vi "main.vi"() -> ()   [LabVIEW 2018]
uses:
  Ctls/LoggingRate.ctl
  Ctls/MotorConfig.ctl
  Ctls/MotroConfigData.ctl
  Ctls/MagType.ctl
  Ctls/QueueData.ctl
  Ctls/State.ctl
  Ctls/CmdData.ctl
  Ctls/ConsumerLoopData.ctl
  Ctls/DisplayIndicator.ctl
  Ctls/DatabaseCmd.ctl
  Siemens S7 TCP v3_3 LV 8_5/Siemens S7 TCP v3_3 LV 8_5/S7 TCP API Library/S7 TCP.lvlib
panel:
  out "Motor#2_Speed":sgl(knob) caption="电机转速RPM" scale=0.0..50.0
  out "Motor#1_Speed":sgl(knob) caption="电机转速RPM" scale=0.05..50.0
  in  "Motor#2_Config":T1 caption="电机2配置"
  in  "Motor#2_Start?":bool caption="电机启动   1"
  in  "Motor#2_Direction":bool caption="电机方向\n正转          反转    1"
  in  "Motor#2_SpeedSet?":bool
  out "Motor#2_Current":dbl caption="电机电流   1" format="%1.1f"
  in  "Motor#2_SpeedSetting":dbl caption="电机速度设定 1" min=0.0 max=0.0 format="%.3f"
  out "Motor#2_Fault?":bool caption="故障指示 1"
  out "Motor#2_Running?":bool caption="电机运行指示"
  out "Motor#2_ConfigData":T2 caption="2#电机配置数据"
  out "Motor#1_ConfigData":T2 caption="1#电机配置数据"
  in  "Motor#1_Config":T1 caption="电机1配置"
  in  "Motor#1_SpeedSet?":bool
  in  "Log Length":i32=50
  in  "Logging Rate":T4=enum."5Hz"
  in  "Motor#3_Direction":bool caption="电机方向\n正转          反转"
  in  "sample interval (ms)":i32=100
  in  "Record":bool
  out "Speed Log to Display":string[][](table)
  out "Data Read":u8[][](array[numeric])
  out "Float Data Valid?":bool[](array[boolean])
  out "Bool Data Valid":bool
  in  "Stop Button":bool
  out "SpeedCurve":T5(graph) caption="实时显示"
  in  "ClearFault?":bool caption="故障复位"
  in  "Motor#3_SpeedSetting":dbl caption="电机速度设定 3" min=0.0 max=0.0 format="%.3g"
  in  "DualControl_Start?":bool caption="联动启动"
  out "Motor#2_Connected?":bool caption="通讯连接"
  out "Motor#1_Fault?":bool caption="故障指示 1"
  out "Motor#1_Running?":bool caption="电机运行指示"
  out "Motor#1_Connected？":bool caption="通讯连接    1"
  out "Motor#1_Current":dbl caption="电机电流   1" format="%1.1f"
  in  "Motor#1_SpeedSetting":dbl caption="电机速度设定 1" min=0.0 max=0.0 format="%.3f"
  in  "Motor#1_Start?":bool caption="电机启动   1"
  in  "Motor#1_Direction":bool caption="电机方向\n正转          反转    1"
  in  "SingleControl?":bool caption="单动            联动"
  # "1#大电机"
  # "2#大电机"
  # "A"
  # "A"
  # "RPS"
  # "RPS"
  # "RPS"
  # "注意：切换励磁请手动更改驱动器参数P50082,\n 当P50082=0时为永磁，P50082=1时为励磁！！"
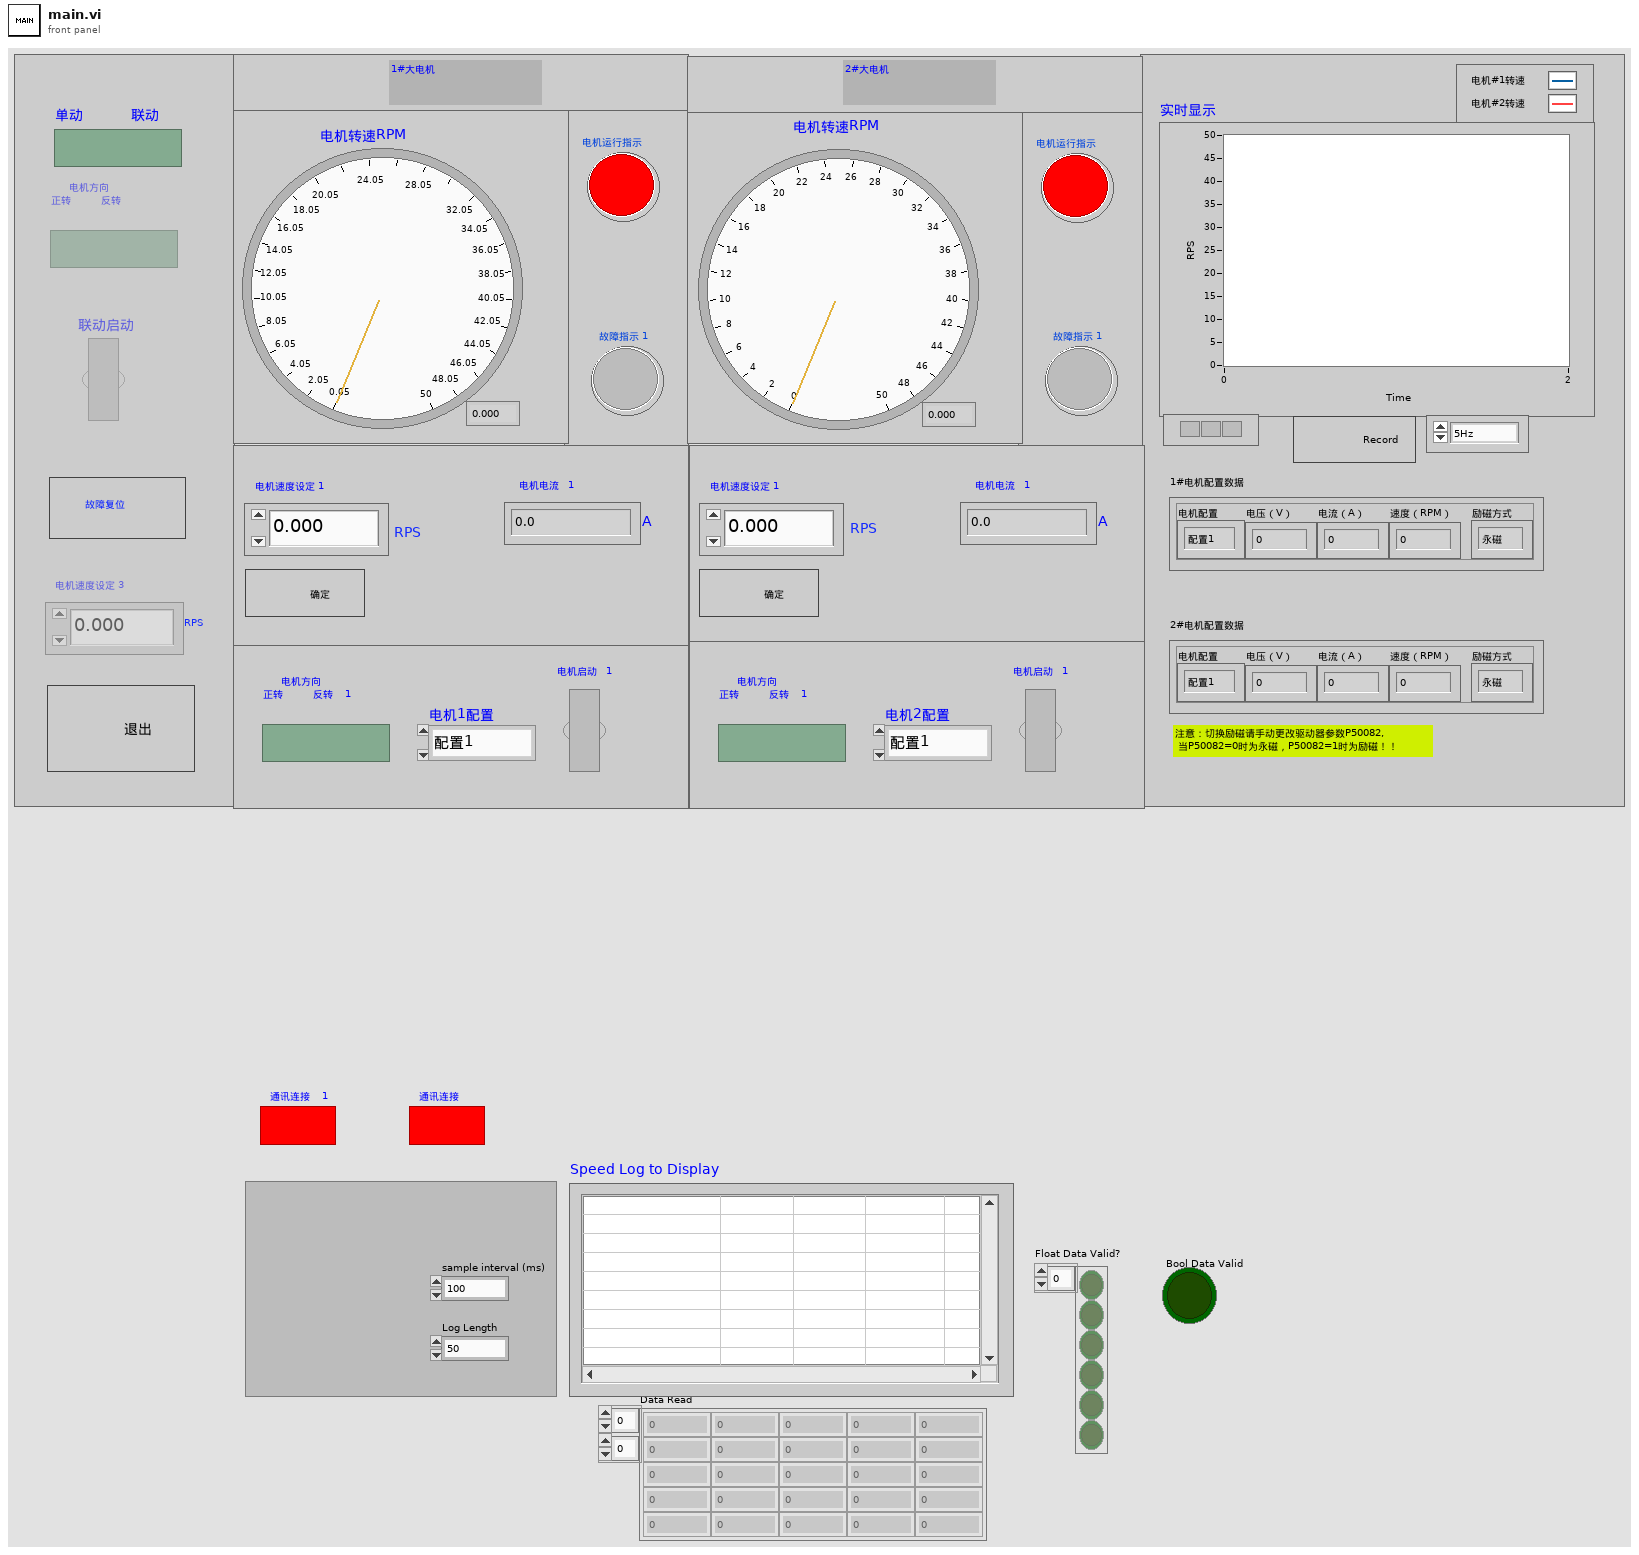
[diagram p1: front panel]
types:
  T1 = typedef "MotorConfig.ctl" = enum16{"配置1", "配置2", "配置3", "配置4"}
  T2 = typedef "MotroConfigData.ctl" = cluster{"电机配置":T1, "电压（V）":dbl, "电流（A）":dbl, "速度（RPM）":dbl, "励磁方式":T3}
  T3 = typedef "MagType.ctl" = enum16{"永磁", "励磁"}
  T4 = typedef "LoggingRate.ctl" = enum16{"1Hz", "2Hz", "5Hz", "10Hz", "20Hz"}
  T5 = cluster{"Motor Speed_1":sgl, "Motor Speed 2":sgl}
  T6 = typedef "ConsumerLoopData.ctl" = cluster{"CmdU16":u16, "Log File Path":path, "PLC Data":T7, "TCP Connection Ref":refnum<k5>, "Config File Path":path}
  T7 = typedef "DisplayIndicator.ctl" = cluster{"CommConnected_1":bool, "Run_1?":bool, "Fault_1?":bool, "CommConnected_2":bool, "Run_2?":bool, "Fault_2?":bool, "Motor Speed 2":sgl, "Motor Speed_1":sgl, "Motor Current_1":sgl, "Motor Current_2":sgl, "Motor1ConfigData":T2, "Motor2ConfigData":T2, "EmoStop_1?":bool}
  T8 = typedef "State.ctl" = enum16{"poll data command", "display update", "init", "send bool command", "send float command", "datalog", "error", "fix rating rpm 1", "fix rating rpm 2", "fix both rating rpm", "fix rating rpm all", "terminate", "log Motor Speed Setting"}
  T9 = typedef "QueueData.ctl" = cluster{"State":T8, "Command Data":T10}
  T10 = typedef "CmdData.ctl" = cluster{"Address Areas":u8, "Data Block #":u16, "Start Address (bytes)":u32, "Write Data Float":sgl, "Bit #":u16, "Write Data Boolean":bool}
  T11 = typedef "DatabaseCmd.ctl" = enum16{"Insert Table Title", "Add One Record", "Delete Record", "Get Table Records", "Clear"}
  T12 = enum8{"Enabled", "Disabled", "Disabled and Grayed Out"}
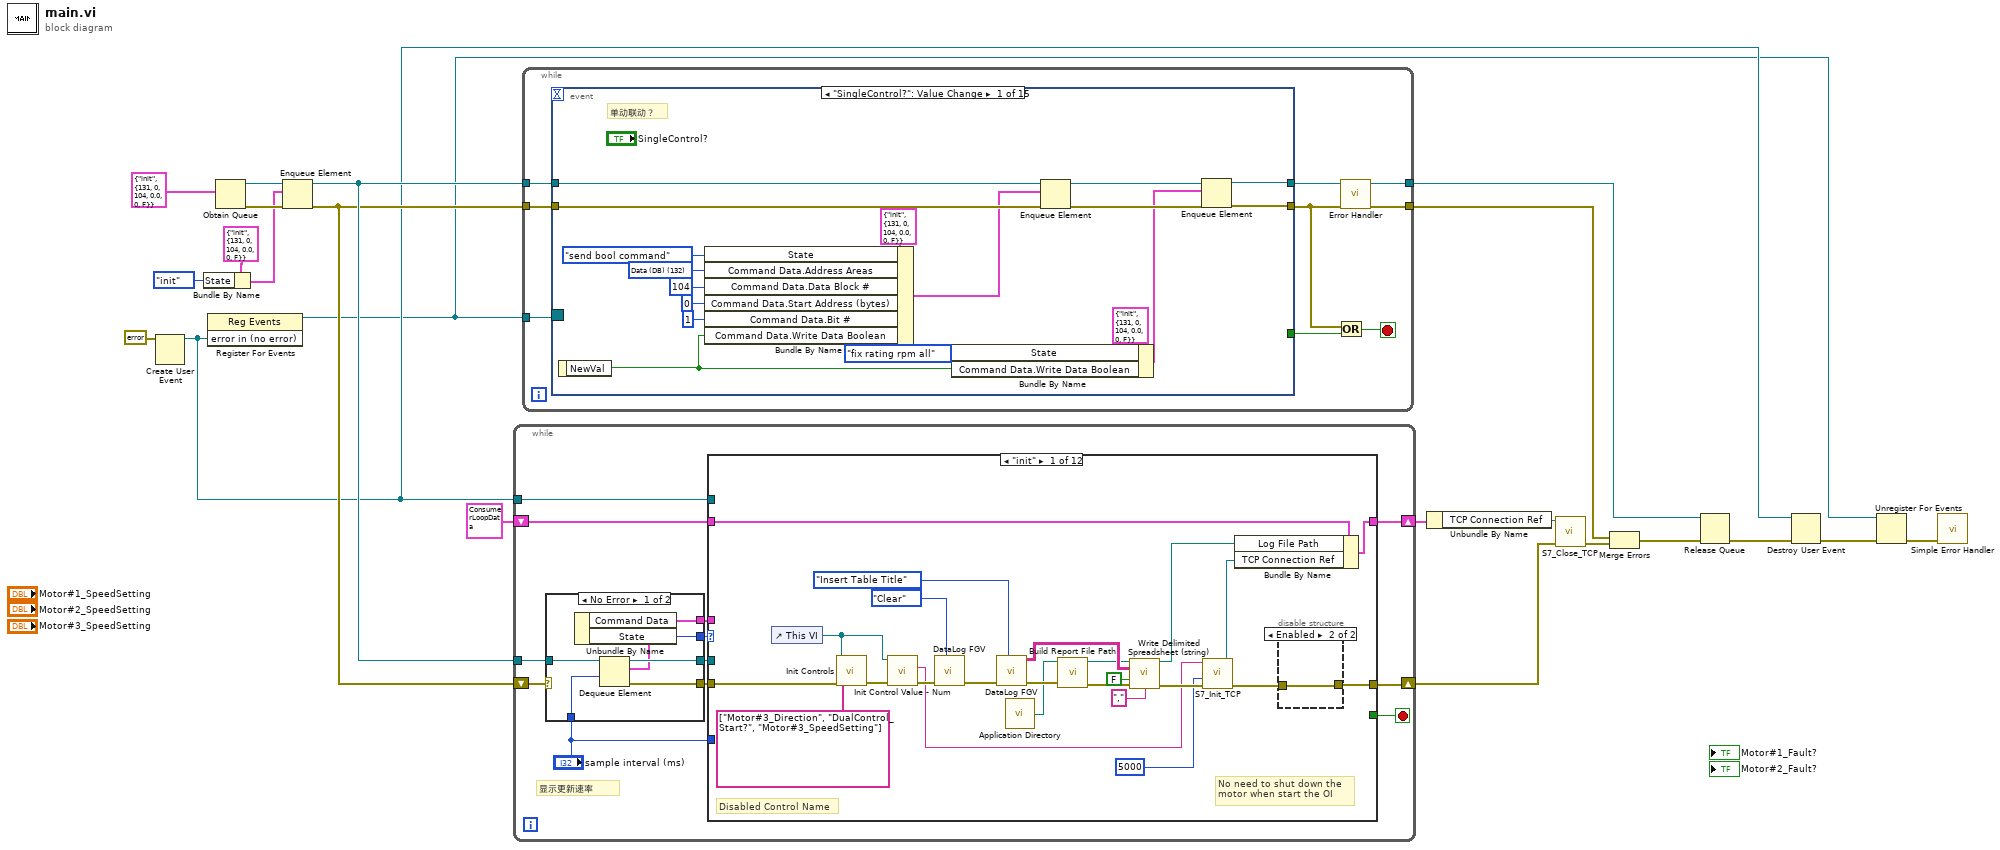
[diagram p0: block diagram]
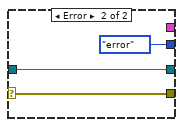
[diagram p2: hidden frame]
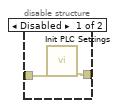
[diagram p3: hidden frame]
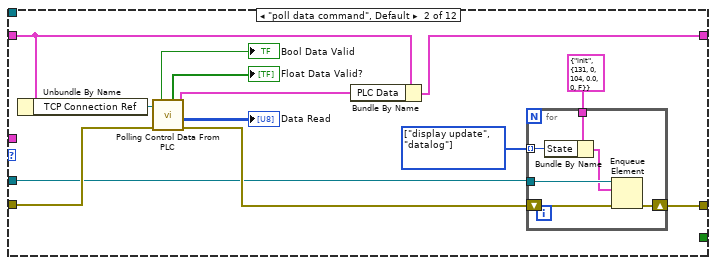
[diagram p4: hidden frame]
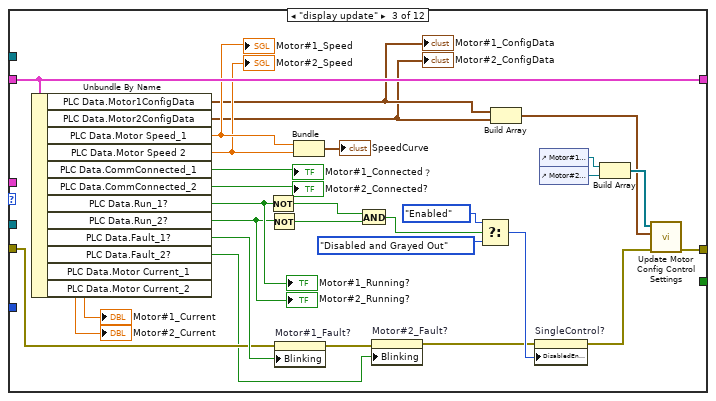
[diagram p5: hidden frame]
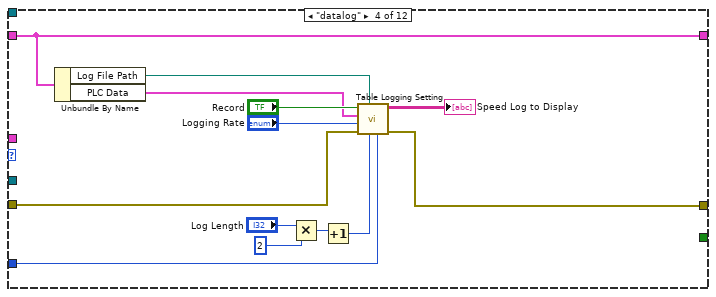
[diagram p6: hidden frame]
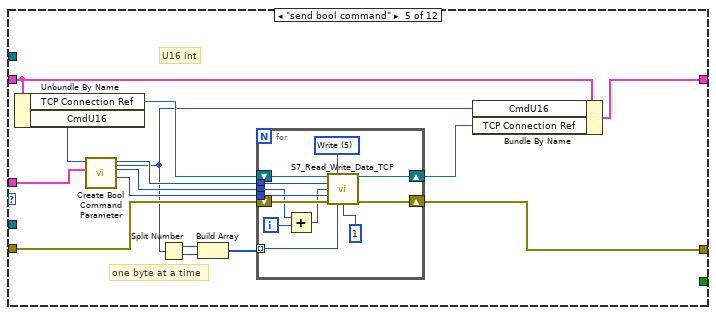
[diagram p7: hidden frame]
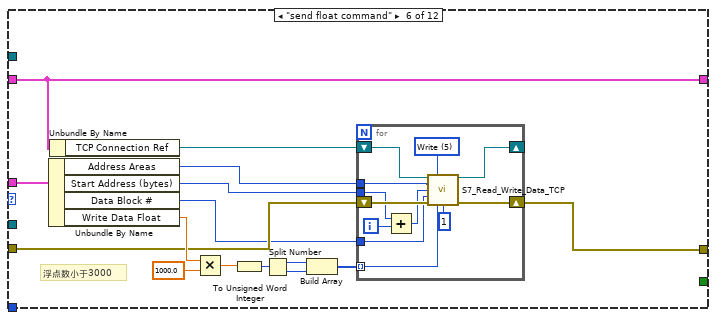
[diagram p8: hidden frame]
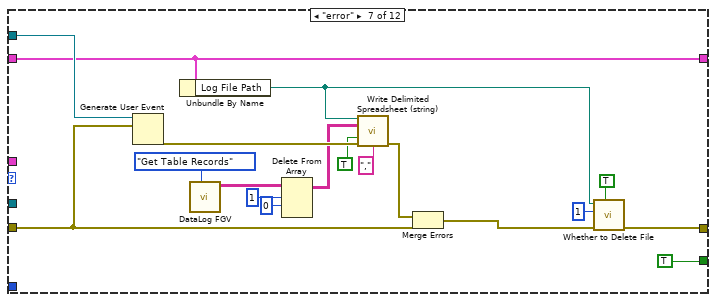
[diagram p9: hidden frame]
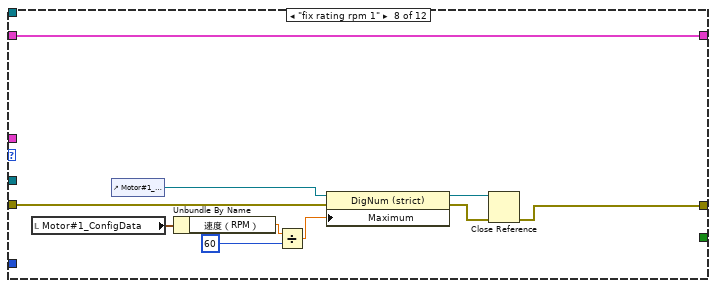
[diagram p10: hidden frame]
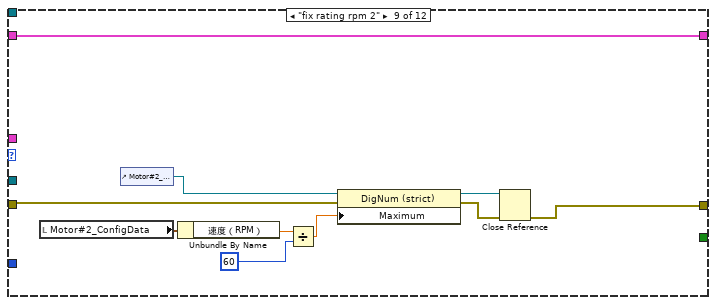
[diagram p11: hidden frame]
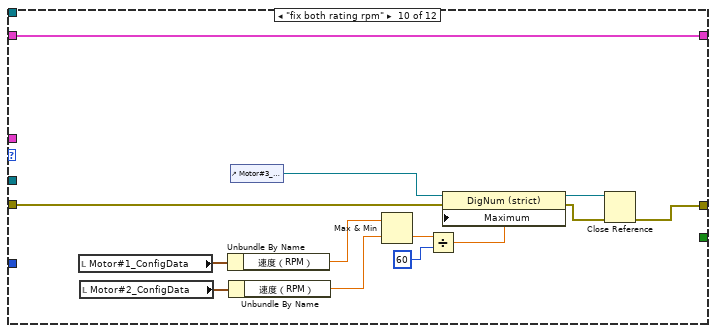
[diagram p12: hidden frame]
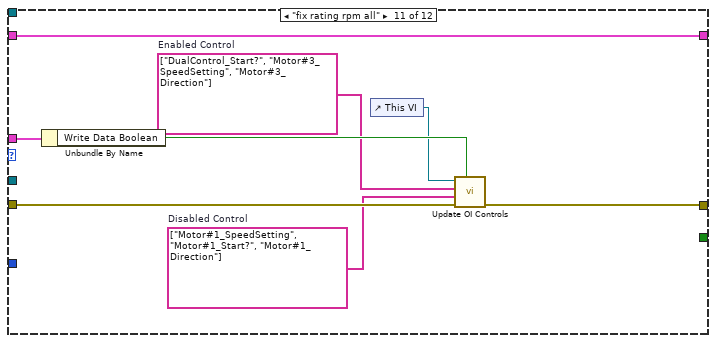
[diagram p13: hidden frame]
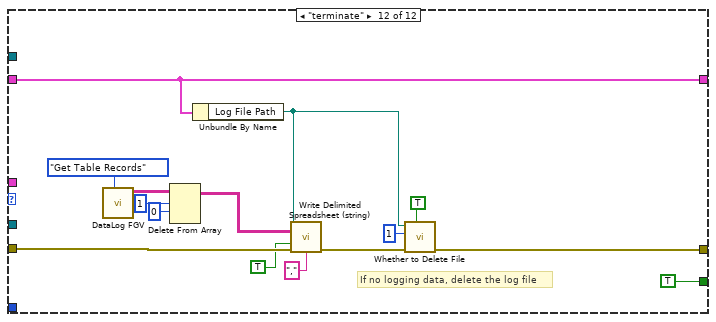
[diagram p14: hidden frame]
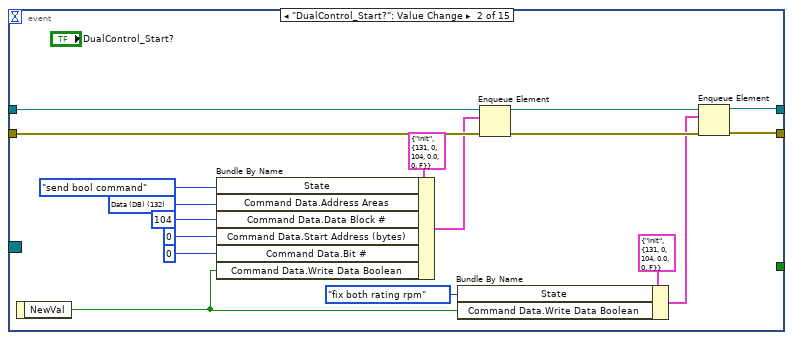
[diagram p15: hidden frame]
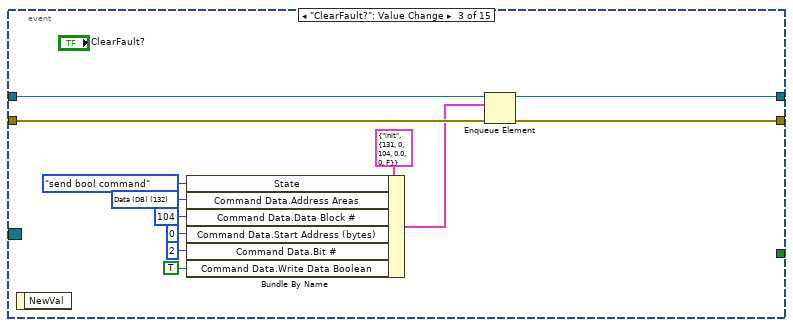
[diagram p16: hidden frame]
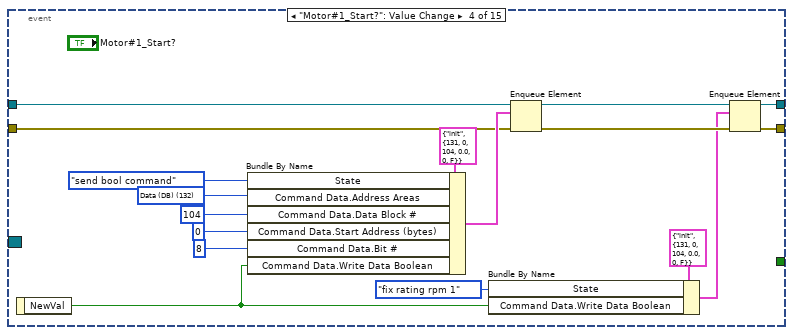
[diagram p17: hidden frame]
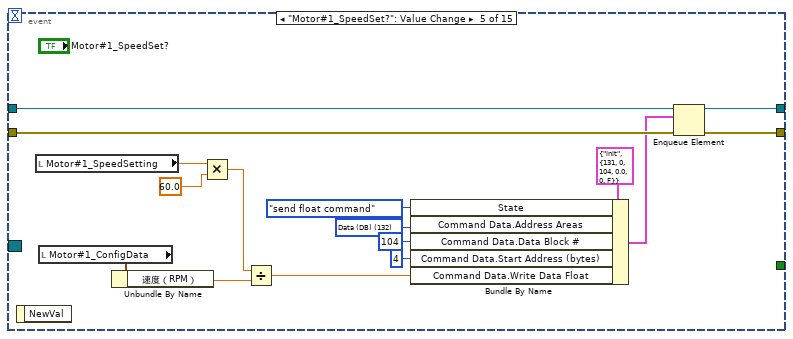
[diagram p18: hidden frame]
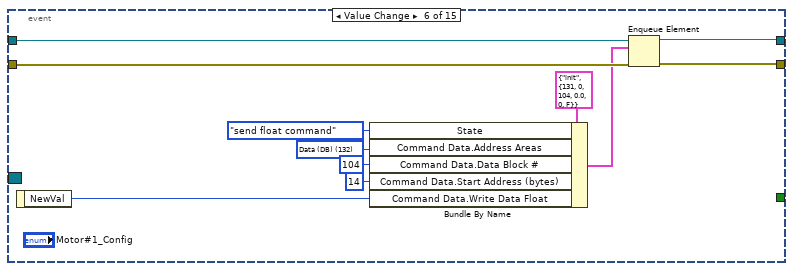
[diagram p19: hidden frame]
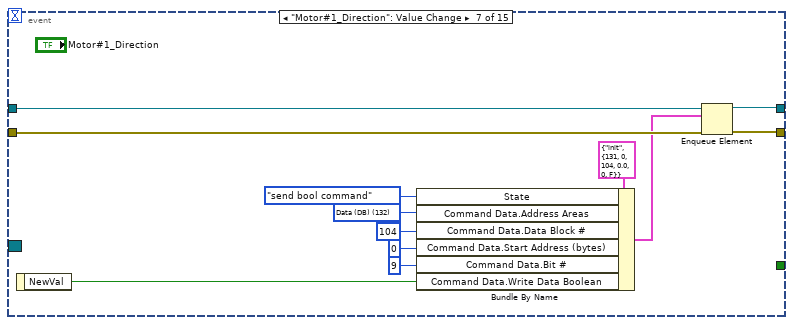
[diagram p20: hidden frame]
diagram:
  n1 = Create User Event(user event datatype=errorcluster {"status"=FALSE, "code"=0, "source"=""} ("error in (no error)")) -> (user event=w13:refnum<user-event>)  [unwired: 1 in, 1 out]
  n2 = Bundle By Name(cluster=T9 {"State"=enum."init", "Command Data"={"Address Areas"=131, "Data Block #"=0, "Start Address (bytes)"=104, "Write Data Float"=0.0, "Bit #"=0, "Write Data Boolean"=FALSE}} ("element"), "State"=State."init") -> (w15:T9)
  n3 = register-events(w13) -> (reference out=w11:refnum<event-registration>)  [unwired: 2 in, 1 out]
  n4 = Obtain Queue(element data type=T9 {"State"=enum."init", "Command Data"={"Address Areas"=131, "Data Block #"=0, "Start Address (bytes)"=104, "Write Data Float"=0.0, "Bit #"=0, "Write Data Boolean"=FALSE}} ("QData")) -> (queue out=w21:refnum<queue>, error out=w19:errorcluster)  [unwired: 4 in, 1 out]
  n5 = Enqueue Element(queue=w21, element=w15, error in (no error)=w19) -> (queue out=w20:refnum<queue>, error out=w18:errorcluster)  [unwired: 1 in, 1 out]
  n6 = while {
    tunnel: w20 -> [w26]
    tunnel: w13 -> [w29]
    shift-right: [w27] -> w10
    shift-left: w18 -> [w28]
    shift-right: [w24] -> w8
    shift-left: T6 {"CmdU16"=0, "Log File Path"=path "", "PLC Data"={"CommConnected_1"=FALSE, "Run_1?"=FALSE, "Fault_1?"=FALSE, "CommConnected_2"=FALSE, "Run_2?"=FALSE, "Fault_2?"=FALSE, "Motor Speed 2"=0.0, "Motor Speed_1"=0.0, "Motor Current_1"=0.0, "Motor Current_2"=0.0, "Motor1ConfigData"={"电机配置"=enum."配置1", "电压（V）"=0.0, "电流（A）"=0.0, "速度（RPM）"=0.0, "励磁方式"=enum."永磁"}, "Motor2ConfigData"={"电机配置"=enum."配置1", "电压（V）"=0.0, "电流（A）"=0.0, "速度（RPM）"=0.0, "励磁方式"=enum."永磁"}, "EmoStop_1?"=FALSE}, "TCP Connection Ref"=refnum, "Config File Path"=path ""} ("Consumer Loop Data") -> [w25]
    stop <- w30 stop-if-true
    # "显示更新速率"
    n7 = case shown="No Error" w28 {
      selector: w28 -> [_ w44]
      tunnel: [w41 w43] -> w34
      tunnel: [w40 w44] -> w33
      tunnel: [w38 State."error" ("State")] -> w32
      tunnel: [w37 _] -> w31
      tunnel: w26 -> [w36 w43]
      tunnel: "sample interval (ms)" -> [w35 _]
      frame No Error {
        n8 = Dequeue Element(queue=w36, timeout in ms (-1)=w35) -> (queue out=w41:refnum<queue>, element=w39:T9, error out=w40:errorcluster)  [unwired: 1 in, 1 out]
        n9 = Unbundle By Name(w39) -> ("Command Data"=w37:T10, "State"=w38:T8)
      }
      frame Error {
      }
    }
    n10 = case shown="\"init\"" w32 {
      tunnel: w34 -> [_ w78 _ _ _ _ _ _ _ _ _ _]
      tunnel: w33 -> [w53 w84 w108 w130 w147 w168 w202 w212 w222 w237 w243 w255]
      tunnel: [w55 w79 w112 w129 w139 w162 w188 w206 w215 w226 w244 w249] -> w27
      tunnel: w31 -> [_ _ _ _ w146 w174 _ _ _ _ w245 _]
      tunnel: [_ _ _ _ _ _ TRUE ("Data Valid") _ _ _ _ TRUE ("Data Valid")] -> w30
      tunnel: w29 -> [_ _ _ _ _ _ w203 _ _ _ _ _]
      tunnel: w25 -> [w52 w75 w111 w121 w136 w160 w192 w205 w216 w225 w242 w251]
      tunnel: [w49 w73 w111 w121 w133 w160 w192 w205 w216 w225 w242 w251] -> w24
      tunnel: "sample interval (ms)" -> [_ _ _ w120 _ _ _ _ _ _ _ _]
      frame "init" {
        # "Disabled Control Name"
        # "No need to shut down the \nmotor when start the OI"
        n11 = control-ref of="This VI"() -> (w46:refnum<vi>)
        n12 = call "Init Controls.vi"("error in"=w53, "Disabled Controls"=string[] ["Motor#3_Direction", "DualControl_Start?", "Motor#3_SpeedSetting"], "VI ref"=w46) -> ("error out"=w48:errorcluster)  [unwired: 8 in]
        n13 = call "Init Control Value - Num.vi"("error in (no error)"=w48, "This VI"=w46) -> ("error out"=w47:errorcluster, "PLC IP"=w45:string)  [unwired: 7 in, 1 out]
        n14 = call "DataLog FGV.vi"("Method"=DatabaseCmd."Clear", "error in (no error)"=w47) -> ("error out"=w68:errorcluster)  [unwired: 7 in, 2 out]
        n15 = call "DataLog FGV.vi"("Method"=DatabaseCmd."Insert Table Title", "error in (no error)"=w68) -> ("error out"=w67:errorcluster, "Speed Log"=w66:string[][])  [unwired: 7 in, 1 out]
        n16 = call <vilib>:"Application Directory.vi"() -> ("Application Directory"=w60:path)
        n17 = call "Build Report File Path.vi"("error in (no error)"=w67, "File Path in"=w60) -> ("error out"=w64:errorcluster, "Report Path out"=w65:path)  [unwired: 8 in]
        n18 = call "Write Delimited Spreadsheet (string).vi"("Path"=w65, "2D data"=w66, "append to file?"=FALSE ("append to file? (new file:F)"), "error in"=w64, "delimiter (\\t)"="," ("delimiter (\\t)")) -> ("path"=w51:path, "error out"=w58:errorcluster)  [unwired: 9 in]
        n19 = call "S7_Init_TCP.vi"("error in"=w58, "Connection Timeout"=u32 5000, "IP Address"=w45) -> ("error out"=w56:errorcluster, "TCP Connection Ref"=w50:refnum<k5>)  [unwired: 2 in, 5 out]
        n20 = Bundle By Name(cluster=w52, "Log File Path"=w51, "TCP Connection Ref"=w50) -> (w49:T6)
        n21 = disable-structure shown="Enabled" {
          disable-tunnel: w56 -> [w70 w71]
          disable-tunnel: [w69 w71] -> w55
          frame Disabled {
            n22 = call "Init PLC Settings.vi"("error in"=w70) -> ("error out"=w69:errorcluster)  [unwired: 9 in, 1 out]
          }
          frame Enabled {
          }
        }
      }
      frame "poll data command", Default {
        w76 = T8[] [enum."display update", enum."datalog"] items=["poll data command", "display update", "init", "send bool command", "send float command", "datalog", "error", "fix rating rpm 1", "fix rating rpm 2", "fix both rating rpm", "fix rating rpm all", "terminate", "log Motor Speed Setting"]
        n23 = Unbundle By Name(w75) -> ("TCP Connection Ref"=w72:refnum<k5>)
        n24 = call "Polling Control Data From PLC.vi"("error in (no error)"=w84, "TCP Network Connection in"=w72) -> ("error out"=w80:errorcluster, "Data Read"=→"Data Read":u8[][], "PLC Data out"=w74:T7, "Bool Data Valid"=→"Bool Data Valid":bool, "Float Data Valid?"=→"Float Data Valid?":bool[])  [unwired: 2 in, 3 out]
        n25 = Bundle By Name(cluster=w75, "PLC Data"=w74) -> (w73:T6)
        n26 = for {
          tunnel: w78 -> [w88]
          shift-right: [w89] -> w79
          shift-left: w80 -> [w90]
          tunnel: T9 {"State"=enum."init", "Command Data"={"Address Areas"=131, "Data Block #"=0, "Start Address (bytes)"=104, "Write Data Float"=0.0, "Bit #"=0, "Write Data Boolean"=FALSE}} ("QData") -> [w86]
          tunnel: w76 -> [w85] mode=indexing
          n27 = Bundle By Name(cluster=w86, "State"=w85) -> (w87:T9)
          n28 = Enqueue Element(queue=w88, element=w87, error in (no error)=w90) -> (error out=w89:errorcluster)  [unwired: 1 in, 2 out]
        }
      }
      frame "display update" {
        n29 = Unbundle By Name(w111) -> ("PLC Data.Motor1ConfigData"=w96:T2, "PLC Data.Motor2ConfigData"=w95:T2, "PLC Data.Motor Speed_1"=w98:sgl, "PLC Data.Motor Speed 2"=w97:sgl, "PLC Data.CommConnected_1"=→"Motor#1_Connected？":bool, "PLC Data.CommConnected_2"=→"Motor#2_Connected?":bool, "PLC Data.Run_1?"=w100:bool, "PLC Data.Run_2?"=w99:bool, "PLC Data.Fault_1?"=w109:bool, "PLC Data.Fault_2?"=w107:bool, "PLC Data.Motor Current_1"=→"Motor#1_Current":sgl, "PLC Data.Motor Current_2"=→"Motor#2_Current":sgl)
        "Motor#1_Running?" <- w100
        "Motor#2_Running?" <- w99
        "Motor#1_ConfigData" <- w96
        "Motor#2_ConfigData" <- w95
        "Motor#1_Speed" <- w98
        "Motor#2_Speed" <- w97
        n30 = Not(x=w100) -> (.not. x?=w118:bool)
        n31 = Not(x=w99) -> (.not. x?=w119:bool)
        n32 = property on="Motor#1_Fault?" class="Bool (strict)"(error in=w108, "Blinking"=w109) -> (error out=w106:errorcluster)  [unwired: 1 in, 1 out]
        n33 = Bundle("Motor Speed_1"=w98, "Motor Speed 2"=w97) -> (→"SpeedCurve":T5)  [unwired: 1 in]
        n34 = And(x=w118, y=w119) -> (x .and. y?=w117:bool)
        n35 = property on="Motor#2_Fault?" class="Bool (strict)"(error in=w106, "Blinking"=w107) -> (error out=w105:errorcluster)  [unwired: 1 in, 1 out]
        n36 = Select(t=T12."Enabled" ("Disabled"), s=w117, f=T12."Disabled and Grayed Out" ("Disabled")) -> (s? t:f=w114:T12)
        n37 = Build Array(w96, w95) -> (w91:T2[])
        n38 = property on="SingleControl?" class="Bool (strict)"(error in=w105, "DisabledEnum"=w114) -> (error out=w113:errorcluster)  [unwired: 1 in, 1 out]
        n39 = control-ref of="Motor#1_Config"() -> (w94:refnum<vi>)
        n40 = control-ref of="Motor#2_Config"() -> (w93:refnum<vi>)
        n41 = Build Array(w94, w93) -> (w92:refnum<vi>[])
        n42 = call "Update Motor Config Control Settings.vi"("error in (no error)"=w113, "Motor Config Data"=w91, "Motor Config Refs"=w92) -> ("error out"=w112:errorcluster)  [unwired: 8 in]
      }
      frame "datalog" {
        n43 = Unbundle By Name(w121) -> ("Log File Path"=w123:path, "PLC Data"=w122:T7)
        n44 = Multiply(x="Log Length", y=2) -> (x*y=w125:i32)
        n45 = Increment(x=w125) -> (x+1=w124:i32)
        n46 = call "Table Logging Setting.vi"("sample interval (ms)"=w120, "Log Length"=w124, "Log File path"=w123, "error in (no error)"=w130, "Logging Rate"="Logging Rate", "Data In"=w122, "Record"="Record") -> ("error out"=w129:errorcluster, "Speed Log to Display"=→"Speed Log to Display":string[][])  [unwired: 3 in]
      }
      frame "send bool command" {
        # "one byte at a time"
        # "U16 int"
        n47 = Unbundle By Name(w136) -> ("TCP Connection Ref"=w137:refnum<k5>, "CmdU16"=w138:u16)
        n48 = call "Create Bool Command Parameter.vi"("Command Data"=w146, "Cmd U16"=w138) -> ("Data Block #"=w143:u16, "Start Address (bytes)"=w144:u32, "Address Areas"=w145:u8, "Cmd U16 out"=w135:u16)  [unwired: 6 in]
        n49 = Split Number(x=w135) -> (hi(x)=w141:u8, lo(x)=w140:u8)
        n50 = Build Array(w141, w140) -> (w142:u8[])
        n51 = for {
          tunnel: w145 -> [w155]
          tunnel: w144 -> [w149]
          tunnel: w143 -> [w154]
          shift-right: [w156] -> w134
          shift-left: w137 -> [w159]
          shift-right: [w152] -> w139
          shift-left: w147 -> [w158]
          tunnel: w142 -> [w151] mode=indexing
          i -> [w150]
          w157 = u8 5 items=["Read"=4, "Write"=5] ("Read / Write")
          n52 = Add(x=w149, y=w150) -> (x+y=w148:u32)
          n53 = call "S7_Read_Write_Data_TCP.vi"("TCP Connection Ref"=w159, "Read / Write"=w157, "Address Areas"=w155, "Start Address (bytes)"=w148, "Data Block #"=w154, "error in"=w158, "Write Data"=w151, "Length (bytes)"=u16 1) -> ("TCP Connection Ref Out"=w156:refnum<k5>, "error out"=w152:errorcluster)  [unwired: 2 in, 4 out]
        }
        n54 = Bundle By Name(cluster=w136, "CmdU16"=w135, "TCP Connection Ref"=w134) -> (w133:T6)
      }
      frame "send float command" {
        # "浮点数小于3000"
        n55 = Unbundle By Name(w174) -> ("Address Areas"=w167:u8, "Start Address (bytes)"=w166:u32, "Data Block #"=w165:u16, "Write Data Float"=w173:sgl)
        n56 = Unbundle By Name(w160) -> ("TCP Connection Ref"=w161:refnum<k5>)
        n57 = Multiply(x=w173, y=sgl 1000.0) -> (x*y=w171:sgl)
        n58 = To Unsigned Word Integer(number=w171) -> (unsigned 16bit integer=w170:u16)
        n59 = Split Number(x=w170) -> (hi(x)=w164:u8, lo(x)=w163:u8)
        n60 = Build Array(w164, w163) -> (w169:u8[])
        n61 = for {
          shift-right: [w183] -> _
          shift-left: w161 -> [w186]
          shift-right: [w181] -> w162
          shift-left: w168 -> [w185]
          tunnel: w169 -> [w178] mode=indexing
          tunnel: w167 -> [w177]
          tunnel: w166 -> [w176]
          tunnel: w165 -> [w175]
          i -> [w180]
          w184 = u8 5 items=["Read"=4, "Write"=5] ("Read / Write")
          n62 = Add(x=w176, y=w180) -> (x+y=w179:u32)
          n63 = call "S7_Read_Write_Data_TCP.vi"("TCP Connection Ref"=w186, "Read / Write"=w184, "Address Areas"=w177, "Start Address (bytes)"=w179, "Data Block #"=w175, "error in"=w185, "Write Data"=w178, "Length (bytes)"=u16 1) -> ("TCP Connection Ref Out"=w183:refnum<k5>, "error out"=w181:errorcluster)  [unwired: 2 in, 4 out]
        }
      }
      frame "error" {
        n64 = Generate User Event(user event=w203, event data cluster=w202) -> (error out=w201:errorcluster)  [unwired: 2 in, 1 out]
        n65 = Unbundle By Name(w192) -> ("Log File Path"=w187:path)
        n66 = call "DataLog FGV.vi"("Method"=DatabaseCmd."Get Table Records") -> ("Speed Log"=w197:string[][])  [unwired: 8 in, 2 out]
        n67 = Delete From Array(array=w197, length=1, index (row)=0) -> (array with subset deleted=w194:string[][])  [unwired: 1 in, 1 out]
        n68 = call "Write Delimited Spreadsheet (string).vi"("Path"=w187, "2D data"=w194, "append to file?"=TRUE ("append to file? (new file:F)"), "error in"=w201, "delimiter (\\t)"="," ("delimiter (\\t)")) -> ("error out"=w200:errorcluster)  [unwired: 9 in, 1 out]
        n69 = Merge Errors(w200, w202) -> (w189:errorcluster)
        n70 = call "Whether to Delete File.vi"("Del Log file?"=TRUE, "error in (no error)"=w189, "Number of lines"=1, "File path"=w187) -> ("error out"=w188:errorcluster)  [unwired: 7 in]
      }
      frame "fix rating rpm 1" {
        n71 = local read "Motor#1_ConfigData"() -> (w208:T2)
        n72 = control-ref of="Motor#1_SpeedSetting"() -> (w211:refnum<vi>)
        n73 = Unbundle By Name(w208) -> ("速度（RPM）"=w207:dbl)
        n74 = Divide(x=w207, y=u16 60) -> (x/y=w213:dbl)
        n75 = property class="DigNum (strict)"(reference=w211, error in=w212, "Maximum"=w213) -> (reference out=w209:refnum<vi>, error out=w210:errorcluster)
        n76 = Close Reference(reference=w209, error in (no error)=w210) -> (error out=w206:errorcluster)
      }
      frame "fix rating rpm 2" {
        n77 = local read "Motor#2_ConfigData"() -> (w219:T2)
        n78 = control-ref of="Motor#2_SpeedSetting"() -> (w217:refnum<vi>)
        n79 = Unbundle By Name(w219) -> ("速度（RPM）"=w218:dbl)
        n80 = Divide(x=w218, y=u16 60) -> (x/y=w223:dbl)
        n81 = property class="DigNum (strict)"(reference=w217, error in=w222, "Maximum"=w223) -> (reference out=w220:refnum<vi>, error out=w221:errorcluster)
        n82 = Close Reference(reference=w220, error in (no error)=w221) -> (error out=w215:errorcluster)
      }
      frame "fix both rating rpm" {
        n83 = local read "Motor#1_ConfigData"() -> (w228:T2)
        n84 = local read "Motor#2_ConfigData"() -> (w230:T2)
        n85 = Unbundle By Name(w228) -> ("速度（RPM）"=w227:dbl)
        n86 = Unbundle By Name(w230) -> ("速度（RPM）"=w229:dbl)
        n87 = control-ref of="Motor#3_SpeedSetting"() -> (w236:refnum<vi>)
        n88 = Max & Min(x=w227, y=w229) -> (min(x,y)=w233:dbl)  [unwired: 1 out]
        n89 = Divide(x=w233, y=u16 60) -> (x/y=w231:dbl)
        n90 = property class="DigNum (strict)"(reference=w236, error in=w237, "Maximum"=w231) -> (reference out=w234:refnum<vi>, error out=w235:errorcluster)
        n91 = Close Reference(reference=w234, error in (no error)=w235) -> (error out=w226:errorcluster)
      }
      frame "fix rating rpm all" {
        w239 = string[] ["DualControl_Start?", "Motor#3_SpeedSetting", "Motor#3_Direction"]  # Enabled Control
        w238 = string[] ["Motor#1_SpeedSetting", "Motor#1_Start?", "Motor#1_Direction"]  # Disabled Control
        n92 = Unbundle By Name(w245) -> ("Write Data Boolean"=w241:bool)
        n93 = control-ref of="This VI"() -> (w240:refnum<vi>)
        n94 = call "Update OI Controls.vi"("ControlBoth?"=w241, "error in (no error)"=w243, "Disabled Controls"=w238, "Enabled Controls"=w239, "VI Ref"=w240) -> ("error out"=w244:errorcluster)  [unwired: 6 in]
      }
      frame "terminate" {
        # "If no logging data, delete the log file"
        n95 = call "DataLog FGV.vi"("Method"=DatabaseCmd."Get Table Records") -> ("Speed Log"=w258:string[][])  [unwired: 8 in, 2 out]
        n96 = Delete From Array(array=w258, length=1, index (row)=0) -> (array with subset deleted=w254:string[][])  [unwired: 1 in, 1 out]
        n97 = Unbundle By Name(w251) -> ("Log File Path"=w248:path)
        n98 = call "Write Delimited Spreadsheet (string).vi"("Path"=w248, "2D data"=w254, "append to file?"=TRUE ("append to file? (new file:F)"), "error in"=w255, "delimiter (\\t)"="," ("delimiter (\\t)")) -> ("error out"=w250:errorcluster)  [unwired: 9 in, 1 out]
        n99 = call "Whether to Delete File.vi"("Del Log file?"=TRUE, "error in (no error)"=w250, "Number of lines"=1, "File path"=w248) -> ("error out"=w249:errorcluster)  [unwired: 7 in]
      }
    }
  }
  n100 = while {
    tunnel: w20 -> [w269]
    tunnel: w18 -> [w268]
    tunnel: w11 -> [w267]
    tunnel: [w262] -> w5
    tunnel: [w261] -> w4
    stop <- w265 stop-if-true
    n101 = event shown="[0] \"SingleControl?\": Value Change" {
      selector: w267 -> [_ _ _ _ _ _ _ _ _ _ _ _ _ _ _]
      dyn-events: _ -> [_ _ _ _ _ _ _ _ _ _ _ _ _ _ _]
      timeout: _ -> [_ _ _ _ _ _ _ _ _ _ _ _ _ _ _]
      tunnel: [_ _ _ _ _ _ _ _ _ _ _ _ _ TRUE ("Stop Button") TRUE ("Stop Button")] -> w266
      tunnel: w269 -> [w286 w302 w315 w324 w347 w358 w370 w397 w409 w421 w437 w449 w466 w470 w479]
      tunnel: w268 -> [w285 w301 w314 w323 w345 w356 w368 w396 w407 w419 w436 w447 w465 w468 w478]
      tunnel: [w278 w296 w310 w322 w346 w357 w369 w390 w408 w420 w435 w448 w461 w475 w479] -> w264
      tunnel: [w276 w294 w311 w321 w344 w355 w367 w388 w406 w418 w434 w446 w462 w474 w478] -> w263
      event "SingleControl?": Value Change {
        w274 = u8 132 items=["I/O (P)"=128, "Input (I)"=129, "Output (Q)"=130, "Bit Memory (M)"=131, "Data (DB)"=132, "Instance Data (DI)"=133, "Local Data (L)"=134, "Predecessor Local Data (VL)"=135] ("Address Areas")
        # "单动联动？"
        n102 = event-data() -> ("NewVal"=w270:bool)  [unwired: 1 in]
        n103 = Bundle By Name(cluster=T9 {"State"=enum."init", "Command Data"={"Address Areas"=131, "Data Block #"=0, "Start Address (bytes)"=104, "Write Data Float"=0.0, "Bit #"=0, "Write Data Boolean"=FALSE}} ("QData"), "State"=State."send bool command", "Command Data.Address Areas"=w274, "Command Data.Data Block #"=u16 104 ("Data Block #"), "Command Data.Start Address (bytes)"=u32 0 ("Start Address (bytes)"), "Command Data.Bit #"=u16 1 ("Bit #"), "Command Data.Write Data Boolean"=w270) -> (w283:T9)
        n104 = Bundle By Name(cluster=T9 {"State"=enum."init", "Command Data"={"Address Areas"=131, "Data Block #"=0, "Start Address (bytes)"=104, "Write Data Float"=0.0, "Bit #"=0, "Write Data Boolean"=FALSE}} ("QData"), "State"=State."fix rating rpm all", "Command Data.Write Data Boolean"=w270) -> (w275:T9)
        n105 = Enqueue Element(queue=w286, element=w283, error in (no error)=w285) -> (queue out=w279:refnum<queue>, error out=w277:errorcluster)  [unwired: 1 in, 1 out]
        n106 = Enqueue Element(queue=w279, element=w275, error in (no error)=w277) -> (queue out=w278:refnum<queue>, error out=w276:errorcluster)  [unwired: 1 in, 1 out]
      }
      event "DualControl_Start?": Value Change {
        w288 = u8 132 items=["I/O (P)"=128, "Input (I)"=129, "Output (Q)"=130, "Bit Memory (M)"=131, "Data (DB)"=132, "Instance Data (DI)"=133, "Local Data (L)"=134, "Predecessor Local Data (VL)"=135] ("Address Areas")
        n107 = event-data() -> ("NewVal"=w287:bool)  [unwired: 1 in]
        n108 = Bundle By Name(cluster=T9 {"State"=enum."init", "Command Data"={"Address Areas"=131, "Data Block #"=0, "Start Address (bytes)"=104, "Write Data Float"=0.0, "Bit #"=0, "Write Data Boolean"=FALSE}} ("QData"), "State"=State."send bool command", "Command Data.Address Areas"=w288, "Command Data.Data Block #"=u16 104 ("Data Block #"), "Command Data.Start Address (bytes)"=u32 0 ("Start Address (bytes)"), "Command Data.Bit #"=u16 0 ("Bit #"), "Command Data.Write Data Boolean"=w287) -> (w300:T9)
        n109 = Bundle By Name(cluster=T9 {"State"=enum."init", "Command Data"={"Address Areas"=131, "Data Block #"=0, "Start Address (bytes)"=104, "Write Data Float"=0.0, "Bit #"=0, "Write Data Boolean"=FALSE}} ("QData"), "State"=State."fix both rating rpm", "Command Data.Write Data Boolean"=w287) -> (w292:T9)
        n110 = Enqueue Element(queue=w302, element=w300, error in (no error)=w301) -> (queue out=w297:refnum<queue>, error out=w295:errorcluster)  [unwired: 1 in, 1 out]
        n111 = Enqueue Element(queue=w297, element=w292, error in (no error)=w295) -> (queue out=w296:refnum<queue>, error out=w294:errorcluster)  [unwired: 1 in, 1 out]
      }
      event "ClearFault?": Value Change {
        w308 = u8 132 items=["I/O (P)"=128, "Input (I)"=129, "Output (Q)"=130, "Bit Memory (M)"=131, "Data (DB)"=132, "Instance Data (DI)"=133, "Local Data (L)"=134, "Predecessor Local Data (VL)"=135] ("Address Areas")
        n112 = event-data() -> ()  [unwired: 1 in, 1 out]
        n113 = Bundle By Name(cluster=T9 {"State"=enum."init", "Command Data"={"Address Areas"=131, "Data Block #"=0, "Start Address (bytes)"=104, "Write Data Float"=0.0, "Bit #"=0, "Write Data Boolean"=FALSE}} ("QData"), "State"=State."send bool command", "Command Data.Address Areas"=w308, "Command Data.Data Block #"=u16 104 ("Data Block #"), "Command Data.Start Address (bytes)"=u32 0 ("Start Address (bytes)"), "Command Data.Bit #"=u16 2 ("Bit #"), "Command Data.Write Data Boolean"=TRUE ("Write Data Boolean")) -> (w313:T9)
        n114 = Enqueue Element(queue=w315, element=w313, error in (no error)=w314) -> (queue out=w310:refnum<queue>, error out=w311:errorcluster)  [unwired: 1 in, 1 out]
      }
      event "Motor#1_Start?": Value Change {
        w320 = u8 132 items=["I/O (P)"=128, "Input (I)"=129, "Output (Q)"=130, "Bit Memory (M)"=131, "Data (DB)"=132, "Instance Data (DI)"=133, "Local Data (L)"=134, "Predecessor Local Data (VL)"=135] ("Address Areas")
        n115 = event-data() -> ("NewVal"=w316:bool)  [unwired: 1 in]
        n116 = Bundle By Name(cluster=T9 {"State"=enum."init", "Command Data"={"Address Areas"=131, "Data Block #"=0, "Start Address (bytes)"=104, "Write Data Float"=0.0, "Bit #"=0, "Write Data Boolean"=FALSE}} ("QData"), "State"=State."send bool command", "Command Data.Address Areas"=w320, "Command Data.Data Block #"=u16 104 ("Data Block #"), "Command Data.Start Address (bytes)"=u32 0 ("Start Address (bytes)"), "Command Data.Bit #"=u16 8 ("Bit #"), "Command Data.Write Data Boolean"=w316) -> (w331:T9)
        n117 = Bundle By Name(cluster=T9 {"State"=enum."init", "Command Data"={"Address Areas"=131, "Data Block #"=0, "Start Address (bytes)"=104, "Write Data Float"=0.0, "Bit #"=0, "Write Data Boolean"=FALSE}} ("QData"), "State"=State."fix rating rpm 1", "Command Data.Write Data Boolean"=w316) -> (w325:T9)
        n118 = Enqueue Element(queue=w324, element=w331, error in (no error)=w323) -> (queue out=w328:refnum<queue>, error out=w327:errorcluster)  [unwired: 1 in, 1 out]
        n119 = Enqueue Element(queue=w328, element=w325, error in (no error)=w327) -> (queue out=w322:refnum<queue>, error out=w321:errorcluster)  [unwired: 1 in, 1 out]
      }
      event "Motor#1_SpeedSet?": Value Change {
        w336 = u8 132 items=["I/O (P)"=128, "Input (I)"=129, "Output (Q)"=130, "Bit Memory (M)"=131, "Data (DB)"=132, "Instance Data (DI)"=133, "Local Data (L)"=134, "Predecessor Local Data (VL)"=135] ("Address Areas")
        n120 = event-data() -> ()  [unwired: 1 in, 1 out]
        n121 = local read "Motor#1_SpeedSetting"() -> (w339:dbl)
        n122 = local read "Motor#1_ConfigData"() -> (w338:T2)
        n123 = Unbundle By Name(w338) -> ("速度（RPM）"=w337:dbl)
        n124 = Multiply(x=w339, y=60.0) -> (x*y=w340:dbl)
        n125 = Divide(x=w340, y=w337) -> (x/y=w333:dbl)
        n126 = Bundle By Name(cluster=T9 {"State"=enum."init", "Command Data"={"Address Areas"=131, "Data Block #"=0, "Start Address (bytes)"=104, "Write Data Float"=0.0, "Bit #"=0, "Write Data Boolean"=FALSE}} ("QData"), "State"=State."send float command", "Command Data.Address Areas"=w336, "Command Data.Data Block #"=u16 104 ("Data Block #"), "Command Data.Start Address (bytes)"=u32 4 ("Start Address (bytes)"), "Command Data.Write Data Float"=w333) -> (w343:T9)
        n127 = Enqueue Element(queue=w347, element=w343, error in (no error)=w345) -> (queue out=w346:refnum<queue>, error out=w344:errorcluster)  [unwired: 1 in, 1 out]
      }
      event Value Change {
        w352 = u8 132 items=["I/O (P)"=128, "Input (I)"=129, "Output (Q)"=130, "Bit Memory (M)"=131, "Data (DB)"=132, "Instance Data (DI)"=133, "Local Data (L)"=134, "Predecessor Local Data (VL)"=135] ("Address Areas")
        n128 = event-data() -> ("NewVal"=w349:T1)  [unwired: 1 in]
        n129 = Bundle By Name(cluster=T9 {"State"=enum."init", "Command Data"={"Address Areas"=131, "Data Block #"=0, "Start Address (bytes)"=104, "Write Data Float"=0.0, "Bit #"=0, "Write Data Boolean"=FALSE}} ("QData"), "State"=State."send float command", "Command Data.Address Areas"=w352, "Command Data.Data Block #"=u16 104 ("Data Block #"), "Command Data.Start Address (bytes)"=u32 14 ("Start Address (bytes)"), "Command Data.Write Data Float"=w349) -> (w354:T9)
        n130 = Enqueue Element(queue=w358, element=w354, error in (no error)=w356) -> (queue out=w357:refnum<queue>, error out=w355:errorcluster)  [unwired: 1 in, 1 out]
      }
      event "Motor#1_Direction": Value Change {
        w364 = u8 132 items=["I/O (P)"=128, "Input (I)"=129, "Output (Q)"=130, "Bit Memory (M)"=131, "Data (DB)"=132, "Instance Data (DI)"=133, "Local Data (L)"=134, "Predecessor Local Data (VL)"=135] ("Address Areas")
        n131 = event-data() -> ("NewVal"=w360:bool)  [unwired: 1 in]
        n132 = Bundle By Name(cluster=T9 {"State"=enum."init", "Command Data"={"Address Areas"=131, "Data Block #"=0, "Start Address (bytes)"=104, "Write Data Float"=0.0, "Bit #"=0, "Write Data Boolean"=FALSE}} ("QData"), "State"=State."send bool command", "Command Data.Address Areas"=w364, "Command Data.Data Block #"=u16 104 ("Data Block #"), "Command Data.Start Address (bytes)"=u32 0 ("Start Address (bytes)"), "Command Data.Bit #"=u16 9 ("Bit #"), "Command Data.Write Data Boolean"=w360) -> (w366:T9)
        n133 = Enqueue Element(queue=w370, element=w366, error in (no error)=w368) -> (queue out=w369:refnum<queue>, error out=w367:errorcluster)  [unwired: 1 in, 1 out]
      }
      event "Motor#3_SpeedSetting": Value Change {
        w377 = u8 132 items=["I/O (P)"=128, "Input (I)"=129, "Output (Q)"=130, "Bit Memory (M)"=131, "Data (DB)"=132, "Instance Data (DI)"=133, "Local Data (L)"=134, "Predecessor Local Data (VL)"=135] ("Address Areas")
        w376 = u8 132 items=["I/O (P)"=128, "Input (I)"=129, "Output (Q)"=130, "Bit Memory (M)"=131, "Data (DB)"=132, "Instance Data (DI)"=133, "Local Data (L)"=134, "Predecessor Local Data (VL)"=135] ("Address Areas")
        # "联机电机速度"
        n134 = event-data() -> ("NewVal"=w394:dbl)  [unwired: 1 in]
        n135 = local read "Motor#1_ConfigData"() -> (w384:T2)
        n136 = Multiply(x=w394, y=60.0) -> (x*y=w392:dbl)
        n137 = Unbundle By Name(w384) -> ("速度（RPM）"=w383:dbl)
        n138 = Divide(x=w392, y=w383) -> (x/y=w372:dbl)
        n139 = local read "Motor#2_ConfigData"() -> (w382:T2)
        n140 = Bundle By Name(cluster=T9 {"State"=enum."init", "Command Data"={"Address Areas"=131, "Data Block #"=0, "Start Address (bytes)"=104, "Write Data Float"=0.0, "Bit #"=0, "Write Data Boolean"=FALSE}} ("QData"), "State"=State."send float command", "Command Data.Address Areas"=w376, "Command Data.Data Block #"=u16 104 ("Data Block #"), "Command Data.Start Address (bytes)"=u32 4 ("Start Address (bytes)"), "Command Data.Write Data Float"=w372) -> (w395:T9)
        n141 = Unbundle By Name(w382) -> ("速度（RPM）"=w381:dbl)
        n142 = Enqueue Element(queue=w397, element=w395, error in (no error)=w396) -> (queue out=w391:refnum<queue>, error out=w389:errorcluster)  [unwired: 1 in, 1 out]
        n143 = Divide(x=w392, y=w381) -> (x/y=w380:dbl)
        n144 = Bundle By Name(cluster=T9 {"State"=enum."init", "Command Data"={"Address Areas"=131, "Data Block #"=0, "Start Address (bytes)"=104, "Write Data Float"=0.0, "Bit #"=0, "Write Data Boolean"=FALSE}} ("QData"), "State"=State."send float command", "Command Data.Address Areas"=w377, "Command Data.Data Block #"=u16 104 ("Data Block #"), "Command Data.Start Address (bytes)"=u32 6 ("Start Address (bytes)"), "Command Data.Write Data Float"=w380) -> (w385:T9)
        n145 = Enqueue Element(queue=w391, element=w385, error in (no error)=w389) -> (queue out=w390:refnum<queue>, error out=w388:errorcluster)  [unwired: 1 in, 1 out]
      }
      event "Motor#3_Direction": Value Change {
        w403 = u8 132 items=["I/O (P)"=128, "Input (I)"=129, "Output (Q)"=130, "Bit Memory (M)"=131, "Data (DB)"=132, "Instance Data (DI)"=133, "Local Data (L)"=134, "Predecessor Local Data (VL)"=135] ("Address Areas")
        n146 = event-data() -> ("NewVal"=w399:bool)  [unwired: 1 in]
        n147 = Bundle By Name(cluster=T9 {"State"=enum."display update", "Command Data"={"Address Areas"=0, "Data Block #"=0, "Start Address (bytes)"=0, "Write Data Float"=0.0, "Bit #"=0, "Write Data Boolean"=FALSE}} ("QData"), "State"=State."send bool command", "Command Data.Address Areas"=w403, "Command Data.Data Block #"=u16 104 ("Data Block #"), "Command Data.Start Address (bytes)"=u32 0 ("Start Address (bytes)"), "Command Data.Bit #"=u16 3 ("Bit #"), "Command Data.Write Data Boolean"=w399) -> (w405:T9)
        n148 = Enqueue Element(queue=w409, element=w405, error in (no error)=w407) -> (queue out=w408:refnum<queue>, error out=w406:errorcluster)  [unwired: 1 in, 1 out]
      }
      event Value Change {
        w415 = u8 132 items=["I/O (P)"=128, "Input (I)"=129, "Output (Q)"=130, "Bit Memory (M)"=131, "Data (DB)"=132, "Instance Data (DI)"=133, "Local Data (L)"=134, "Predecessor Local Data (VL)"=135] ("Address Areas")
        n149 = event-data() -> ("NewVal"=w412:T1)  [unwired: 1 in]
        n150 = Bundle By Name(cluster=T9 {"State"=enum."init", "Command Data"={"Address Areas"=131, "Data Block #"=0, "Start Address (bytes)"=104, "Write Data Float"=0.0, "Bit #"=0, "Write Data Boolean"=FALSE}} ("QData"), "State"=State."send float command", "Command Data.Address Areas"=w415, "Command Data.Data Block #"=u16 104 ("Data Block #"), "Command Data.Start Address (bytes)"=u32 16 ("Start Address (bytes)"), "Command Data.Write Data Float"=w412) -> (w411:T9)
        n151 = Enqueue Element(queue=w421, element=w411, error in (no error)=w419) -> (queue out=w420:refnum<queue>, error out=w418:errorcluster)  [unwired: 1 in, 1 out]
      }
      event "Motor#2_SpeedSet?": Value Change {
        w425 = u8 132 items=["I/O (P)"=128, "Input (I)"=129, "Output (Q)"=130, "Bit Memory (M)"=131, "Data (DB)"=132, "Instance Data (DI)"=133, "Local Data (L)"=134, "Predecessor Local Data (VL)"=135] ("Address Areas")
        n152 = event-data() -> ()  [unwired: 1 in, 1 out]
        n153 = local read "Motor#2_SpeedSetting"() -> (w432:dbl)
        n154 = local read "Motor#2_ConfigData"() -> (w431:T2)
        n155 = Unbundle By Name(w431) -> ("速度（RPM）"=w430:dbl)
        n156 = Multiply(x=w432, y=60.0) -> (x*y=w433:dbl)
        n157 = Divide(x=w433, y=w430) -> (x/y=w429:dbl)
        n158 = Bundle By Name(cluster=T9 {"State"=enum."init", "Command Data"={"Address Areas"=131, "Data Block #"=0, "Start Address (bytes)"=104, "Write Data Float"=0.0, "Bit #"=0, "Write Data Boolean"=FALSE}} ("QData"), "State"=State."send float command", "Command Data.Address Areas"=w425, "Command Data.Data Block #"=u16 104 ("Data Block #"), "Command Data.Start Address (bytes)"=u32 6 ("Start Address (bytes)"), "Command Data.Write Data Float"=w429) -> (w422:T9)
        n159 = Enqueue Element(queue=w437, element=w422, error in (no error)=w436) -> (queue out=w435:refnum<queue>, error out=w434:errorcluster)  [unwired: 1 in, 1 out]
      }
      event "Motor#2_Direction": Value Change {
        w444 = u8 132 items=["I/O (P)"=128, "Input (I)"=129, "Output (Q)"=130, "Bit Memory (M)"=131, "Data (DB)"=132, "Instance Data (DI)"=133, "Local Data (L)"=134, "Predecessor Local Data (VL)"=135] ("Address Areas")
        n160 = event-data() -> ("NewVal"=w440:bool)  [unwired: 1 in]
        n161 = Bundle By Name(cluster=T9 {"State"=enum."init", "Command Data"={"Address Areas"=131, "Data Block #"=0, "Start Address (bytes)"=104, "Write Data Float"=0.0, "Bit #"=0, "Write Data Boolean"=FALSE}} ("QData"), "State"=State."send bool command", "Command Data.Address Areas"=w444, "Command Data.Data Block #"=u16 104 ("Data Block #"), "Command Data.Start Address (bytes)"=u32 0 ("Start Address (bytes)"), "Command Data.Bit #"=u16 11 ("Bit #"), "Command Data.Write Data Boolean"=w440) -> (w439:T9)
        n162 = Enqueue Element(queue=w449, element=w439, error in (no error)=w447) -> (queue out=w448:refnum<queue>, error out=w446:errorcluster)  [unwired: 1 in, 1 out]
      }
      event "Motor#2_Start?": Value Change {
        w456 = u8 132 items=["I/O (P)"=128, "Input (I)"=129, "Output (Q)"=130, "Bit Memory (M)"=131, "Data (DB)"=132, "Instance Data (DI)"=133, "Local Data (L)"=134, "Predecessor Local Data (VL)"=135] ("Address Areas")
        n163 = event-data() -> ("NewVal"=w450:bool)  [unwired: 1 in]
        n164 = Bundle By Name(cluster=T9 {"State"=enum."init", "Command Data"={"Address Areas"=131, "Data Block #"=0, "Start Address (bytes)"=104, "Write Data Float"=0.0, "Bit #"=0, "Write Data Boolean"=FALSE}} ("QData"), "State"=State."send bool command", "Command Data.Address Areas"=w456, "Command Data.Data Block #"=u16 104 ("Data Block #"), "Command Data.Start Address (bytes)"=u32 0 ("Start Address (bytes)"), "Command Data.Bit #"=u16 10 ("Bit #"), "Command Data.Write Data Boolean"=w450) -> (w452:T9)
        n165 = Bundle By Name(cluster=T9 {"State"=enum."init", "Command Data"={"Address Areas"=131, "Data Block #"=0, "Start Address (bytes)"=104, "Write Data Float"=0.0, "Bit #"=0, "Write Data Boolean"=FALSE}} ("QData"), "State"=State."fix rating rpm 2", "Command Data.Write Data Boolean"=w450) -> (w451:T9)
        n166 = Enqueue Element(queue=w466, element=w452, error in (no error)=w465) -> (queue out=w464:refnum<queue>, error out=w463:errorcluster)  [unwired: 1 in, 1 out]
        n167 = Enqueue Element(queue=w464, element=w451, error in (no error)=w463) -> (queue out=w461:refnum<queue>, error out=w462:errorcluster)  [unwired: 1 in, 1 out]
      }
      event "Stop Button": Value Change {
        n168 = event-data() -> ()  [unwired: 1 in, 1 out]
        n169 = call "Init PLC Settings.vi"("error in"=w468, "queue in"=w470) -> ("error out"=w467:errorcluster, "queue out"=w469:refnum<queue>)  [unwired: 8 in]
        n170 = Bundle By Name(cluster=T9 {"State"=enum."init", "Command Data"={"Address Areas"=131, "Data Block #"=0, "Start Address (bytes)"=104, "Write Data Float"=0.0, "Bit #"=0, "Write Data Boolean"=FALSE}} ("QData"), "State"=State."terminate") -> (w472:T9)
        n171 = Enqueue Element(queue=w469, element=w472, error in (no error)=w467) -> (queue out=w475:refnum<queue>, error out=w474:errorcluster)  [unwired: 1 in, 1 out]
      }
      event User Event {
        n172 = event-data() -> ()  [unwired: 1 in, 1 out]
      }
    }
    n173 = Or(x=w263, y=w266) -> (x .or. y?=w265:bool)
    n174 = call "Error Handler.vi"("error in (no error)"=w263, "queue in"=w264) -> ("error out"=w262:errorcluster, "queue out"=w261:refnum<queue>)  [unwired: 8 in]
  }
  n175 = Unbundle By Name(w8) -> ("TCP Connection Ref"=w7:refnum<k5>)
  n176 = call "S7_Close_TCP.vi"("error in"=w10, "TCP Connection Ref"=w7) -> ("error out"=w6:errorcluster)  [unwired: 1 in, 8 out]
  n177 = Merge Errors(w5, w6) -> (w3:errorcluster)
  n178 = Release Queue(queue=w4, error in (no error)=w3) -> (error out=w2:errorcluster)  [unwired: 1 in, 2 out]
  n179 = Destroy User Event(user event=w13, error in=w2) -> (error out=w12:errorcluster)
  n180 = Unregister For Events(event registration refnum=w11, error in=w12) -> (error out=w1:errorcluster)
  n181 = call <vilib>:"Simple Error Handler.vi"("error in (no error)"=w1) -> ()  [unwired: 4 in, 5 out]
